vi "CLD 17 GUI number pad solution.vi"(8 "Fehler (Eingang, kein Fehler)":errorcluster) -> (0 "Fehler (Ausgang)":errorcluster, 3 "Numerisch":dbl)   [LabVIEW 2014]
doc: "CLD-Übung 17\n\nDieses VI reagiert mit Hilfe einer Polling-Methode auf die Änderungen der GUI. Der Tastenindex basiert auf der Tabulatorreihenfolge des typdefinierten Elements. Mit der Case-Struktur \"Aktionsauswahl\" kann die Anwendung später erweitert werden."
uses:
  CLD 17 Keypad_Typedef.ctl
panel:
  out "String":string="0"
  in  "Keypad-Cluster":T1
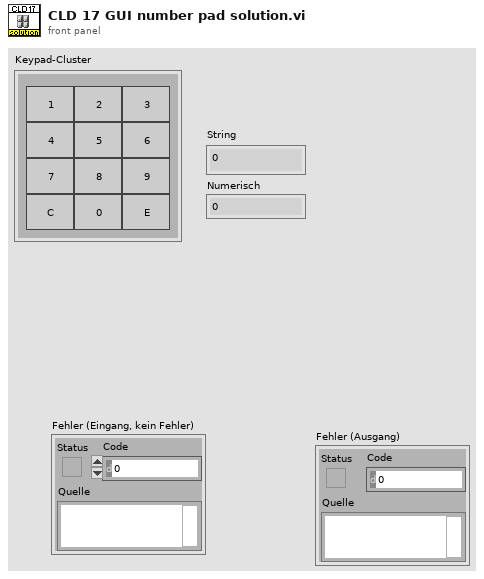
[diagram p1: front panel]
types:
  T1 = typedef "CLD 17 Keypad_Typedef.ctl" = cluster{"0":bool, "1":bool, "2":bool, "3":bool, "4":bool, "5":bool, "6":bool, "7":bool, "8":bool, "9":bool, "C":bool, "E":bool}
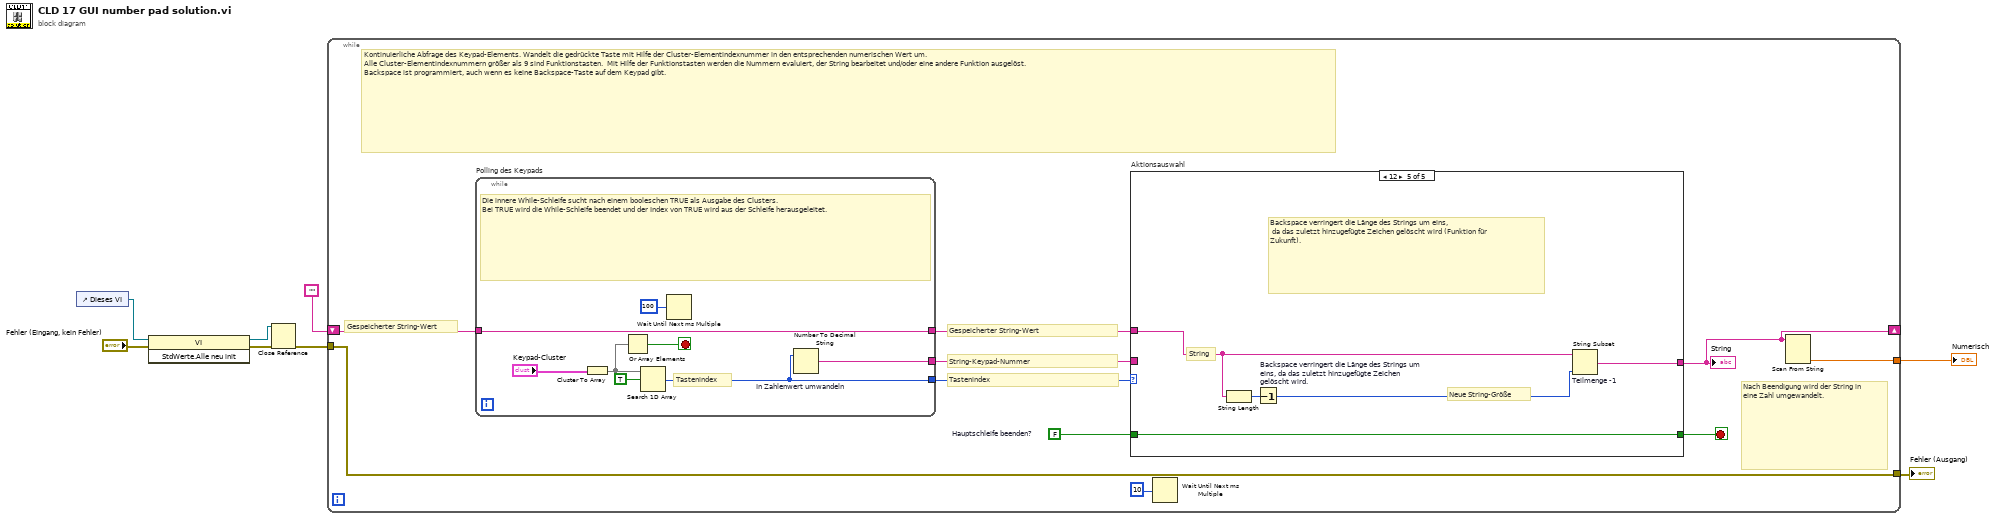
[diagram p0: block diagram]
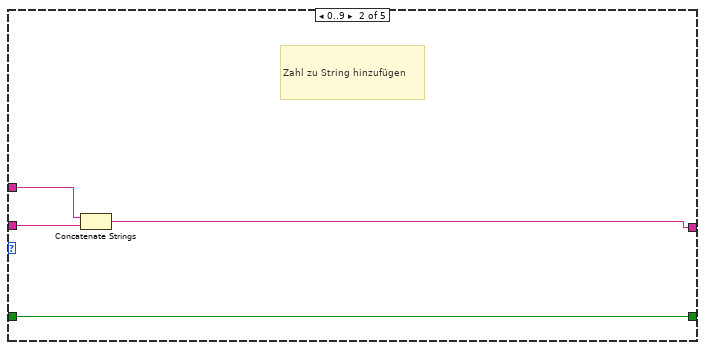
[diagram p3: hidden frame]
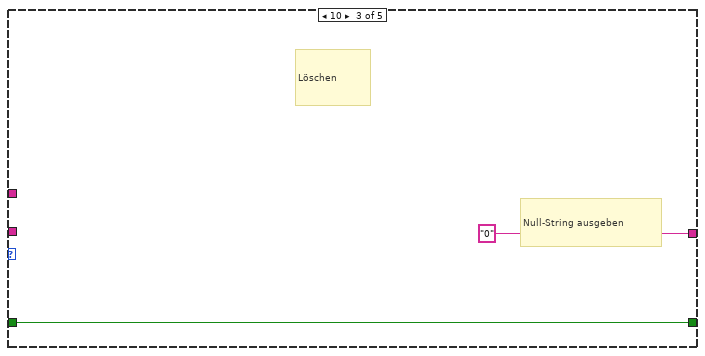
[diagram p4: hidden frame]
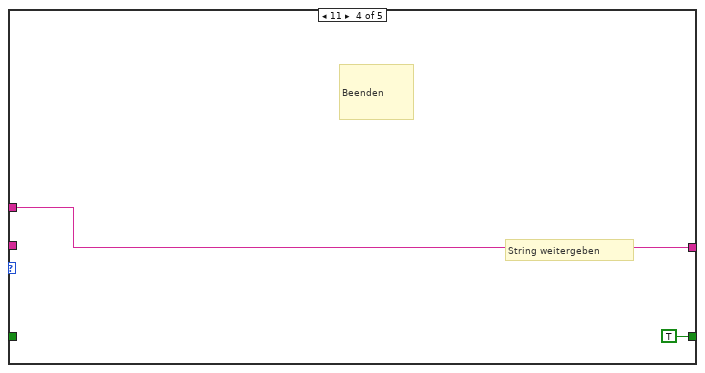
[diagram p5: hidden frame]
diagram:
  n1 = control-ref of="Dieses VI"() -> (w7:refnum<vi>)
  n2 = invoke on="Invoke Node" class="VI" method="StdWerte.Alle neu init"(reference=w7, error in="Fehler (Eingang, kein Fehler)") -> (reference out=w4:refnum<vi>, error out=w6:errorcluster)  [unwired: 1 in, 1 out]
  n3 = Close Reference(reference=w4, error in (no error)=w6) -> (error out=w5:errorcluster)
  n4 = while {
    shift-right: [w14] -> _
    shift-left: "" ("Leerer String (Konstante)") -> [w11]
    tunnel: w5 -> [w9]
    tunnel: [w18] -> w3
    tunnel: [w9] -> w1
    stop <- w13 stop-if-true
    w12 = FALSE  # Hauptschleife beenden?
    # "Nach Beendigung wird der String in eine Zahl umgewandelt."
    # "Kontinuierliche Abfrage des Keypad-Elements. Wandelt die gedrückte Taste mit Hilfe der Cluster-Elementindexnummer in den entsprechenden numerischen Wert um. \nAlle Cluster-Elementindexnummern größer als 9 sind Funktionstasten.  Mit Hilfe der Funktionstasten werden die Nummern evaluiert, der String bearbeitet und/oder eine andere Funktion ausgelöst.  \nBackspace ist programmiert, auch wenn es keine Backspace-Taste auf dem Keypad gibt."
    # "Tastenindex"
    # "String-Keypad-Nummer"
    # "Gespeicherter String-Wert"
    # "Gespeicherter String-Wert"
    n5 = while "Polling des Keypads" {
      tunnel: [w36] -> w16
      tunnel: [w35] -> w15
      tunnel: [w34] -> w10
      tunnel: w11 -> [w34]
      stop <- w38 stop-if-true
      # "Tastenindex"
      # "Die innere While-Schleife sucht nach einem booleschen TRUE als Ausgabe des Clusters.\nBei TRUE wird die While-Schleife beendet und der Index von TRUE wird aus der Schleife herausgeleitet."
      n6 = Cluster To Array(cluster="Keypad-Cluster") -> (array=w39:bool[])
      n7 = Or Array Elements(Boolean array=w39) -> (logical OR=w38:bool)
      n8 = Search 1D Array(1D array=w39, element=TRUE ("Element")) -> (index of element=w36:i32)  [unwired: 1 in]
      n9 = Wait Until Next ms Multiple(millisecond multiple=u32 100 ("Vielfache von ms")) -> ()  [unwired: 1 out]
      n10 = Number To Decimal String "In Zahlenwert umwandeln"(number=w36) -> (decimal integer string=w35:string)  [unwired: 1 in]
    }
    n11 = case "Aktionsauswahl" shown="12" w16 {
      tunnel: w10 -> [w20 w24 _ w28 w30]
      tunnel: w15 -> [_ w23 _ _ _]
      tunnel: [w20 w22 "0" w28 w31] -> w14
      tunnel: [w19 w21 w26 TRUE w29] -> w13
      tunnel: w12 -> [w19 w21 w26 _ w29]
      frame Default {
        # "String weitergeben"
      }
      frame 0..9 {
        # "Zahl zu String hinzufügen"
        n12 = Concatenate Strings(w24, w23) -> (w22:string)
      }
      frame 10 {
        # "Null-String ausgeben"
        # "Löschen"
      }
      frame 11 {
        # "String weitergeben"
        # "Beenden"
      }
      frame 12 {
        # "Neue String-Größe"
        # "String"
        # "Backspace verringert die Länge des Strings um eins,\n da das zuletzt hinzugefügte Zeichen gelöscht wird (Funktion für Zukunft)."
        n13 = String Length(string=w30) -> (length=w33:i32)
        n14 = Decrement "Backspace verringert die Länge des Strings um eins, da das zuletzt hinzugefügte Zeichen gelöscht wird."(x=w33) -> (x-1=w32:i32)
        n15 = String Subset "Teilmenge -1"(string=w30, length (rest)=w32) -> (substring=w31:string)  [unwired: 1 in]
      }
    }
    "String" <- w14
    n16 = Wait Until Next ms Multiple(millisecond multiple=u32 10 ("Vielfache von ms")) -> ()  [unwired: 1 out]
    n17 = Scan From String(input string=w14) -> (output 1=w18:dbl)  [unwired: 4 in, 3 out]
  }
  "Numerisch" <- w3
  "Fehler (Ausgang)" <- w1
